vi "dfd_Unbundle Lattice Coef Cluster.vi"(8 "error in (no error)":errorcluster, 11 "Lattice coef":T3) -> (0 "error out":errorcluster, 2 "filter coef out":T1)   [LabVIEW 2017, in "NI_DigFilterLicensed.lvlib"]
uses:
  <vilib>/addons/Digital Filter Design/NI_DigFilterLicensed.lvlib
  <vilib>/addons/Digital Filter Design/_Objects.llb/DFD Filter Structure Type Selector.ctl
  <vilib>/addons/Digital Filter Design/_Objects.llb/DFD Filter Coef.ctl
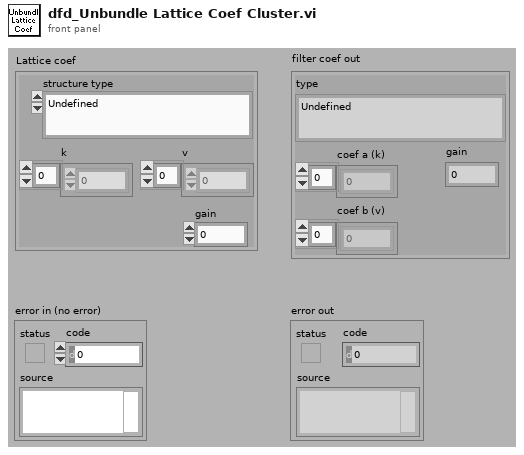
[diagram p1: front panel]
types:
  T1 = typedef "NI_DigFilterLicensed.lvlib/DFD Filter Coef.ctl" = cluster{"type":T2, "gain":dbl, "coef a (k)":dbl[], "coef b (v)":dbl[]}
  T2 = typedef "NI_DigFilterLicensed.lvlib/DFD Filter Structure Type Selector.ctl" = enum16{"Undefined", "FIR Direct Form", "FIR Direct Form Transposed", "FIR Symmetric", "FIR Antisymmetric", "IIR Direct Form I", "IIR Direct Form I Transposed", "IIR Direct Form II", "IIR Direct Form II Transposed", "IIR Cascaded Second Order Sections Form I", "IIR Cascaded Second Order Sections Form I Transposed", "IIR Cascaded Second Order Sections Form II", "IIR Cascaded Second Order Sections Form II Transposed", "Lattice Allpass (basic sections)", "Lattice Allpass (one multiplier sections)", "Lattice Allpass (normalized sections)", "Lattice AR (basic sections)", "Lattice AR (one multiplier sections)", "Lattice AR (normalized sections)", "Lattice MA (minimum phase)", "Lattice MA (maximum phase)", "Lattice ARMA (basic sections)", "Lattice ARMA (one multiplier sections)", "Lattice ARMA (normalized sections)"}
  T3 = cluster{"structure type":T2, "k":dbl[], "v":dbl[], "gain":dbl}
  T4 = enum16{"Undefined", "Basic", "One Multiplier", "Normalized"}
  T5 = typedef "NI_DigFilterLicensed.lvlib/DFD Lattice Type.ctl" = enum16{"Undefined", "Lattice Allpass", "Lattice AR", "Lattice MA (min)", "Lattice MA (max)", "Lattice ARMA"}
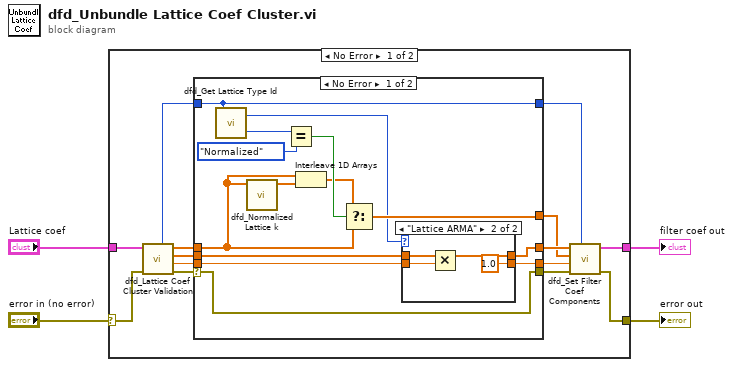
[diagram p0: block diagram]
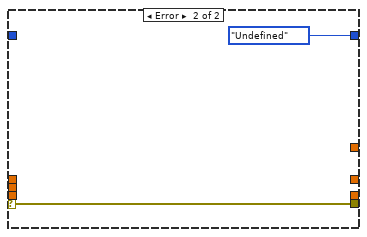
[diagram p3: hidden frame]
diagram:
  n1 = case shown="No Error" "error in (no error)" {
    selector: "error in (no error)" -> [w17 w41]
    tunnel: [w8 w41] -> w3
    tunnel: "Lattice coef" -> [w18 _]
    tunnel: [w9 _] -> w1
    frame No Error {
      n2 = call <vilib>:"dfd_Lattice Coef Cluster Validation.vi"("error in (no error)"=w17, "Lattice coef"=w18) -> ("error out"=w16:errorcluster, "gain"=w12:dbl, "v"=w13:dbl[], "k"=w14:dbl[], "lattice type"=w15:T2)  [unwired: 5 out]
      n3 = case shown="No Error" w16 {
        selector: w16 -> [w32 w40]
        tunnel: [w32 w40] -> w11
        tunnel: w15 -> [w31 _]
        tunnel: w14 -> [w26 _]
        tunnel: w13 -> [w22 _]
        tunnel: w12 -> [w21 _]
        tunnel: [w31 DFD_Filter_Structure_Type_Selector."Undefined" ("structure type")] -> w10
        tunnel: [w24 _] -> w5
        tunnel: [w20 _] -> w7
        tunnel: [w19 _] -> w6
        frame No Error {
          n4 = call <vilib>:"dfd_Get Lattice Type Id.vi"("structure type"=w31) -> ("lattice type"=w23:T5, "section type"=w30:T4)
          n5 = call <vilib>:"dfd_Normalized Lattice k.vi"("k"=w26) -> ("^k"=w28:dbl[])  [unwired: 10 out]
          n6 = Equal?(x=w30, y=T4."Normalized" ("section type")) -> (x = y?=w27:bool)
          n7 = Interleave 1D Arrays(w26, w28) -> (w25:dbl[])
          n8 = Select(t=w25, s=w27, f=w26) -> (s? t:f=w24:dbl[])
          n9 = case shown="\"Lattice ARMA\"" w23 {
            tunnel: w22 -> [w34 w38]
            tunnel: w21 -> [w33 w37]
            tunnel: [w34 w36] -> w19
            tunnel: [w33 1.0 ("gain")] -> w20
            frame "Undefined", Default {
            }
            frame "Lattice ARMA" {
              n10 = Multiply(x=w38, y=w37) -> (x*y=w36:dbl[])
            }
          }
        }
        frame Error {
        }
      }
      n11 = call <vilib>:"dfd_Set Filter Coef Components.vi"("type"=w10, "error in (no error)"=w11, "gain"=w7, "coef a (k)"=w5, "coef b (v)"=w6) -> ("error out"=w8:errorcluster, "filter coef"=w9:T1)  [unwired: 5 out]
    }
    frame Error {
    }
  }
  "error out" <- w3
  "filter coef out" <- w1
